vi "Generate Process DVR.vi"(8 "Error In":errorcluster, 11 "Process In":refnum<class "Process.lvclass">) -> (0 "Error Out":errorcluster, 3 "Process Out":refnum<class "Process.lvclass">)   [LabVIEW 2019, in "Process.lvclass"]
uses:
  Process.lvclass
  Controls/Data.ctl
  Public/Controls/Process Message.ctl
  Central Message Handler/Public/Controls/Message.ctl
  Process.lvclass/Process.ctl
  Central Message Handler/Central Message Handler.lvclass
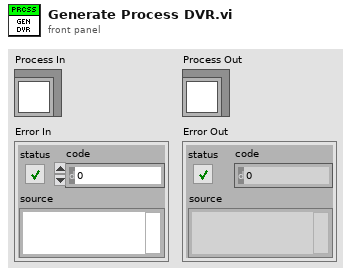
[diagram p1: front panel]
types:
  T1 = typedef "Process.lvclass/Data.ctl" = cluster{"Message Queue":refnum<queue>, "Central Message Queue":refnum<queue>}
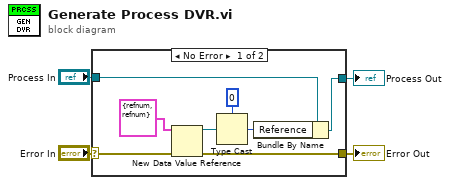
[diagram p0: block diagram]
diagram:
  n1 = case shown="No Error" "Error In" {
    selector: "Error In" -> [w12 w14]
    tunnel: "Process In" -> [w9 w13]
    tunnel: [w8 w13] -> w2
    tunnel: [w7 w14] -> w1
    frame No Error {
      n2 = New Data Value Reference(data value=T1 {"Message Queue"=refnum, "Central Message Queue"=refnum} ("Data"), error in=w12) -> (data value reference=w11:refnum<data-value>, error out=w7:errorcluster)
      n3 = Type Cast(type=u64 0, x=w11) -> (*(type *) &x=w6:u64)
      n4 = Bundle By Name(cluster=w9, "Reference"=w6) -> (w8:refnum<class "Process.lvclass">)
    }
    frame Error {
    }
  }
  "Error Out" <- w1
  "Process Out" <- w2
